vi "Measure Cursors.vi"(0 "Instrument Handle In":i32, 11 "error in":errorcluster) -> (3 "Delta Magnitude":dbl, 4 "Instrument Handle Out":i32, 6 "Cursor1 Time":dbl, 8 "Cursor1 Magnitude":dbl, 10 "Cursor2 Time":dbl, 13 "Delta Time":dbl, 14 "Cursor2 Magnitude":dbl, 15 "error out":errorcluster)   [LabVIEW 8.6, in "ZTScopeM.lvlib"]
doc: "This function gets the cursors' measurement data."
uses:
  ZTScopeM.lvlib
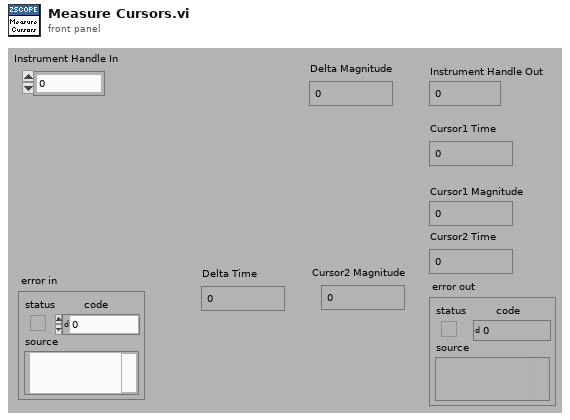
[diagram p1: front panel]
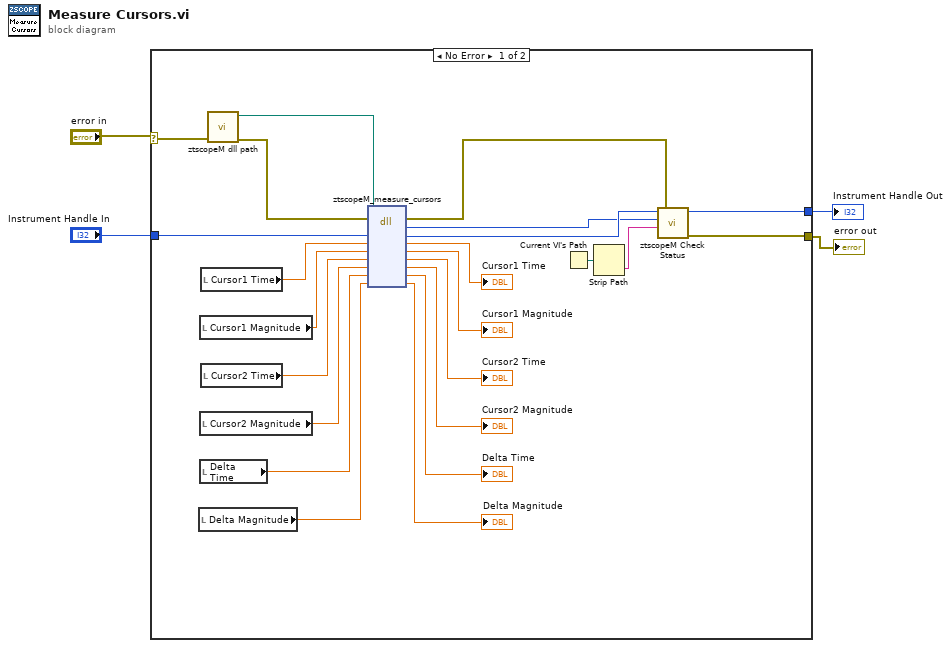
[diagram p0: block diagram]
diagram:
  n1 = case shown="No Error" "error in" {
    selector: "error in" -> [w8 w29]
    tunnel: [w10 w29] -> w1
    tunnel: "Instrument Handle In" -> [w27 w28]
    tunnel: [w9 w28] -> w3
    frame #0 {
      n2 = local read "Delta Magnitude"() -> (w16:dbl)
      n3 = local read "Cursor1 Magnitude"() -> (w24:dbl)
      n4 = local read "Cursor2 Magnitude"() -> (w20:dbl)
      n5 = local read "Delta Time"() -> (w18:dbl)
      n6 = local read "Cursor1 Time"() -> (w26:dbl)
      n7 = local read "Cursor2 Time"() -> (w22:dbl)
      n8 = call "ztscopeM dll path.vi"("error in (no error)"=w8) -> ("error out"=w6:errorcluster, "<instrument>.dll path"=w7:path)  [unwired: 9 in]
      n9 = dll-call lib="C:/Program Files (x86)/National Instruments/LabVIEW 2013/instr.lib/ztscopem/ztscopeM.dll" fn="ztscopeM_measure_cursors"(path in=w7, error in=w6, "instrumentHandle"=w27, "cursor1Time"=w26, "cursor1Magnitude"=w24, "cursor2Time"=w22, "cursor2Magnitude"=w20, "deltaTime"=w18, "deltaMagnitude"=w16) -> (error out=w5:errorcluster, w11:i32, "instrumentHandle"=w12:i32, "cursor1Time"=→"Cursor1 Time":dbl, "cursor1Magnitude"=→"Cursor1 Magnitude":dbl, "cursor2Time"=→"Cursor2 Time":dbl, "cursor2Magnitude"=→"Cursor2 Magnitude":dbl, "deltaTime"=→"Delta Time":dbl, "deltaMagnitude"=→"Delta Magnitude":dbl)  [unwired: 1 in, 1 out]
      n10 = Current VI's Path() -> (path=w14:path)
      n11 = Strip Path(path=w14) -> (name=w13:string)  [unwired: 1 out]
      n12 = call "ztscopeM Check Status.vi"("error in"=w5, "name of VI"=w13, "status (return code)"=w11, "instrument handle in"=w12) -> ("error out"=w10:errorcluster, "instrument handle out"=w9:i32)  [unwired: 2 in]
    }
    frame #1 {
    }
  }
  "Instrument Handle Out" <- w3
  "error out" <- w1
